vi "TSM DAQmx N Pins To M Tasks.vi"(0 "TSM context":T3, 5 "Pins":tag[](array[tag]), 7 "Site Numbers":i32[](array[numeric]), 11 "error in":errorcluster) -> (4 "DAQ TSM Out":T1, 15 "error out":errorcluster)   [LabVIEW 2019]
doc: "Populates the TSM SSC DAQmx cluster for the specified pin(s) and pin group(s)."
uses:
  <vilib>/NI_TestStand_SemiconductorModule/NI_TestStand_Semiconductor_Module.lvlibp/PinMap/General/SemiconductorModuleContext.ctl
  TSM DAQmx Multi-Task.ctl
  <vilib>/NI_TestStand_SemiconductorModule/NI_TestStand_Semiconductor_Module.lvlibp/PinMap/PinQueryContext/MultiplePinMultipleSessionQueryContext/MultiplePinMultipleSessionQueryContext.lvclass
  SSC DAQmx.ctl
  <vilib>/NI_TestStand_SemiconductorModule/NI_TestStand_Semiconductor_Module.lvlibp/PinMap/DAQmx/PinsToNIDAQmxTasks.vi
  <vilib>/NI_TestStand_SemiconductorModule/NI_TestStand_Semiconductor_Module.lvlibp
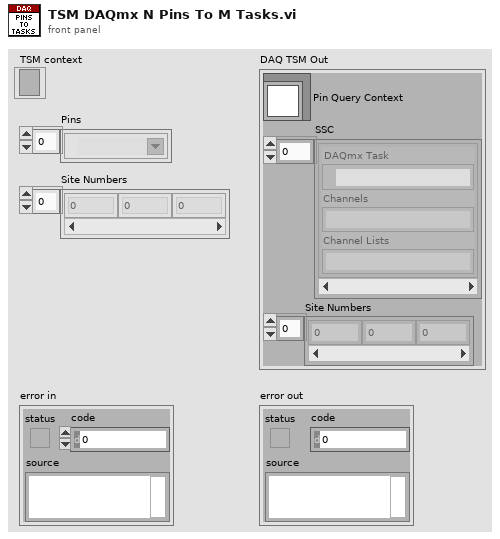
[diagram p1: front panel]
types:
  T1 = typedef "TSM DAQmx Multi-Task.ctl" = cluster{"Pin Query Context":refnum<class "MultiplePinMultipleSessionQueryContext.lvclass">, "SSC":T2[], "Site Numbers":i32[]}
  T2 = typedef "SSC DAQmx.ctl" = cluster{"DAQmx Task ":refnum<k21>, "Channels":string, "Channel Lists":string}
  T3 = typedef "NI_TestStand_Semiconductor_Module.lvlibp/SemiconductorModuleContext.ctl" = refnum<k7>
  T4 = cluster{"DAQmx Task":refnum<k21>, "Channel List":string, "spreadsheet string":string}[]
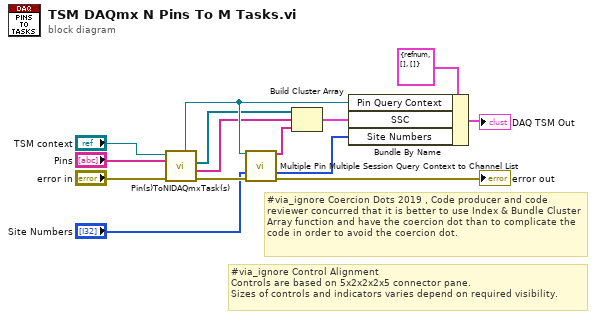
[diagram p0: block diagram]
diagram:
  # "#via_ignore Coercion Dots 2019 , Code producer and code reviewer concurred that it is better to use Index & Bundle Cluster Array function and have the coercion dot than to complicate the code in order to avoid the coercion dot."
  # "#via_ignore Control Alignment\nControls are based on 5x2x2x2x5 connector pane.\nSizes of controls and indicators varies depend on required visibility."
  n1 = call-poly <vilib>:"Pin(s)ToNIDAQmxTask(s).vi"("error in (no error)"="error in", "Pins"="Pins", "Semiconductor Module Context"="TSM context") -> ("error out"=w12:errorcluster, "Channel Lists"=w3:string[], "DAQmx Tasks"=w4:refnum<k21>[], "Pin Query Context"=w5:refnum<class "MultiplePinMultipleSessionQueryContext.lvclass">)  [unwired: 4 in, 1 out]
  n2 = call "Multiple Pin Multiple Session Query Context to Channel List.vi"("Multiple Pin Multiple Sessions Query Context"=w5, "Site Numbers In"="Site Numbers", "error in"=w12) -> ("Per-Session Channel List"=w2:string[], "Site Numbers Out"=w7:i32[], "error out"=→"error out":errorcluster)  [unwired: 10 in]
  n3 = Build Cluster Array(w4, w3, w2) -> (w1:T4)
  n4 = Bundle By Name(cluster=T1 {"Pin Query Context"=refnum, "SSC"=[], "Site Numbers"=[]} ("DAQmx - Multiple Sessions Info"), "Pin Query Context"=w5, "SSC"=w1, "Site Numbers"=w7) -> (→"DAQ TSM Out":T1)
